vi "Advanced 429 Functions.vi"() -> ()   [LabVIEW 2019]
doc: "This program demonstrates the use of advanced 429 protocol features via the configuration file. These features include adjusting signal amplitude, setting bit rate to values other than 12.5 KHz and 100 KHz, adjusting rise and fall times to non-standard values, and channel \"leg lifting\" which allows the positive or negative legs of the signal to be open or shorted to ground rather than the 429 signal. These settings can be combined to perform multiple adjustments at once to different parameters, this is not shown in this example.\n\nThese functions are only available on NI part numbers containing a 45x module (where x is currently 4 or 8).\n\nThe use of these features requires the switching of the active configuration file for the channel. To accomplish this, select a different configuration file in the \"Channel Configuration XML file name\", stop the example if it is currently running, then start the example again."
uses:
  <instrlib>/BTICardLib/Private/Initialize By Card Number and Core Number.vi
  <instrlib>/BTICardLib/Private/Configure Core From XML.vi
  <instrlib>/BTI429Lib/Private/Tx/Configure/Configure Tx Channel From XML.vi
  <instrlib>/BTI429Lib/Private/Core/Action-Status/Start Channel.vi
  <instrlib>/BTI429Lib/Private/Core/Action-Status/Stop Channel.vi
  <instrlib>/BTICardLib/BTICardLV.lvlib
  <instrlib>/BTI429Lib/BTI429LV.lvlib
panel:
  in  "Channel Configuration XML file name":string(combo)="normal.xml"
  out "core number":i32
  out "channel number":i32=8
  in  "Core Configuration XML file name":string="Core Config.xml"
  out "error out":errorcluster
  in  "stop":bool
  in  "Card Number":i32
  # "ARINC 429: Advanced 429 Functions"
  # "©2017 Astronics Ballard Technology"
  # "This program demonstrates the use of advanced 429 protocol features via the configuration file. These features include adjusting signal amplitude, setting bit rate to values other than 12.5 KHz and 100 KHz, adjusting rise and fall times to non-standard values, and channel \"leg lifting\" which allows the positive or negative legs of the signal to be open or shorted to ground rather than the 429 signal. These settings can be combined to perform multiple adjustments at once to different parameters, this is not shown in this example.\n\nThese functions are only available on NI part numbers containing a 45x module (where x is currently 4 or 8).\n\nThe use of these features requires the switching of the active configuration file for the channel. To accomplish this, select a different configuration file in the \"Channel Configuration XML file name\", stop the example if it is currently running, then start the example again."
  # "Always Stop the card\nand Close the card when\ndone. Otherwise, the hardware\ncontinues to operate."
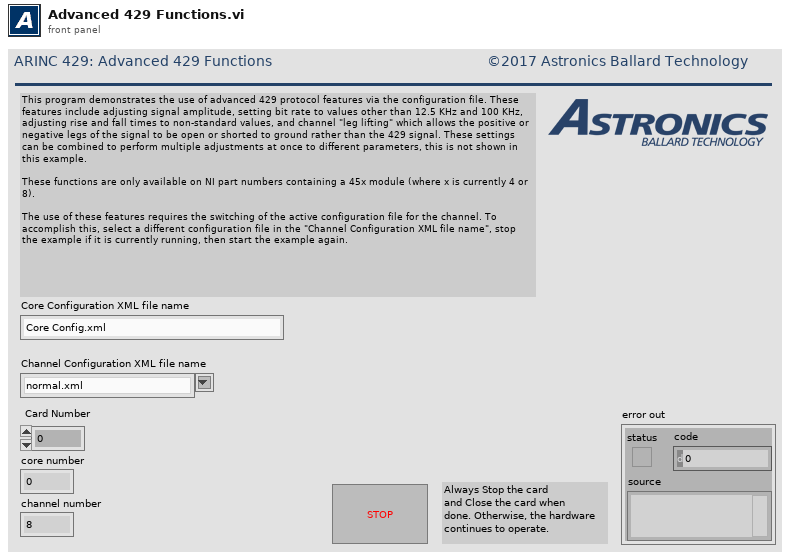
[diagram p1: front panel]
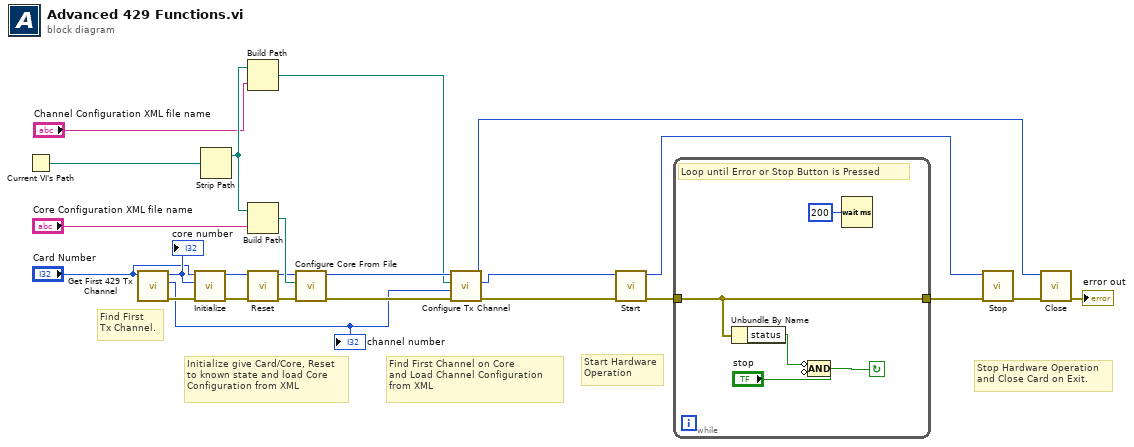
[diagram p0: block diagram]
diagram:
  # "Find First\nTx Channel."
  # "Stop Hardware Operation\nand Close Card on Exit."
  # "Start Hardware\nOperation"
  # "Find First Channel on Core\nand Load Channel Configuration\nfrom XML"
  # "Initialize give Card/Core, Reset\nto known state and load Core\nConfiguration from XML"
  n1 = Current VI's Path() -> (path=w16:path)
  n2 = call "Get First 429 Tx Channel.vi"("Card Number"="Card Number") -> ("error out"=w5:errorcluster, "Channel Number"=w4:i32, "Core Number"=w7:i32)  [unwired: 8 in]
  "channel number" <- w4
  "core number" <- w7
  n3 = call-poly <instrlib>:"Initialize.vi"("error in (no error)"=w5, "core number"=w7, "card number"="Card Number") -> ("error out"=w10:errorcluster, "core handle out"=w11:u64)  [unwired: 7 in]
  n4 = Strip Path(path=w16) -> (stripped path=w14:path)  [unwired: 1 out]
  n5 = Build Path(base path=w14, name or relative path="Channel Configuration XML file name") -> (appended path=w15:path)
  n6 = Build Path(base path=w14, name or relative path="Core Configuration XML file name") -> (appended path=w12:path)
  n7 = call <instrlib>:"Reset.vi"("error in (no error)"=w10, "core handle in"=w11) -> ("error out"=w8:errorcluster, "core handle out"=w9:u64)  [unwired: 8 in]
  n8 = call-poly <instrlib>:"Configure Core From File.vi"("error in (no error)"=w8, "configuration file path"=w12, "core handle in"=w9) -> ("error out"=w21:errorcluster, "core handle out"=w20:u64)  [unwired: 7 in]
  n9 = call-poly <instrlib>:"Configure Tx Channel.vi"("error in (no error)"=w21, "channel number in"=w4, "configuration file path"=w15, "core handle in"=w20) -> ("error out"=w1:errorcluster, "channel handle out"=w2:u64, "core handle out"=w22:u64)  [unwired: 5 in]
  n10 = call-poly <instrlib>:"Start.vi"("error in (no error)"=w1, "channel handle in"=w2) -> ("error out"=w24:errorcluster, "channel handle out"=w19:u64)  [unwired: 8 in]
  n11 = while {
    tunnel: [w25] -> w18
    tunnel: w24 -> [w25]
    stop <- w27 continue-if-true
    # "Loop until Error or Stop Button is Pressed"
    n12 = Unbundle By Name(w25) -> ("status"=w28:bool)
    n13 = Compound Arithmetic op=AND(invert w28, invert "stop") -> (w27:bool)
    n14 = Wait (ms)(milliseconds to wait=u32 200) -> ()  [unwired: 1 out]
  }
  n15 = call-poly <instrlib>:"Stop.vi"("error in (no error)"=w18, "channel handle in"=w19) -> ("error out"=w17:errorcluster)  [unwired: 8 in, 1 out]
  n16 = call <instrlib>:"Close.vi"("error in (no error)"=w17, "core handle in"=w22) -> ("error out"=→"error out":errorcluster)  [unwired: 8 in, 1 out]
